vi "Module Not Stopped--error.vi"() -> (0 "error out":errorcluster)   [LabVIEW 2018, in "6509.lvlib"]
doc: "Outputs an error cluster containing a custom error code indicating the Stop Module VI timed out while waiting for the module main VI to stop.\n_____\nBased on Delacor QMH Project Template 4.2.1.64."
uses:
  6509.lvlib
  <vilib>/Utility/error.llb/Error Cluster From Error Code.vi
  <vilib>/ErrorRing/Error Ring.xnode
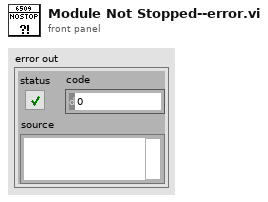
[diagram p1: front panel]
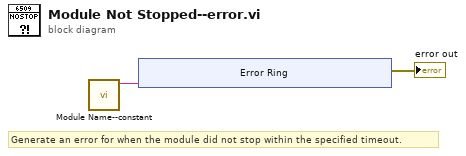
[diagram p0: block diagram]
diagram:
  # "Generate an error for when the module did not stop within the specified timeout."
  n1 = call "Module Name--constant.vi"() -> ("Module Name"=w1:string)  [unwired: 11 in]
  n2 = xnode "Error Ring"("parameter 0"=w1) -> ("error out"=→"error out":errorcluster)
